vi "ReadWord.vi"(7 "Adresse":T1, 8 "error in (no error)":errorcluster, 9 "Parameter [0 ... 65535]":u16, 10 "Befehl [0 ... 65535]":u16, 11 "VISA resource name":refnum<visa-resource-name>) -> (0 "error out":errorcluster, 1 "Read Buffer":string, 2 "Regler Rückgabewert [0 ... 65535]":u16, 3 "VISA resource name out":refnum<visa-resource-name>)   [LabVIEW 2023, in "TCxxxx.lvlib"]
doc: "This VI reads a WORD value from the TCxxxx device.\n\n\nInput:\n\n- Adresse [ENUM]: this is the adress at which the function performs the read\n- Befehl [UINT16]: this is the command to the device.\n- Parameter [UINT16]: this is the parameter to read from the device (unused, always set to 0)\n\n\nOutput:\n\n- Regler Rückgabewert [UINT16]: this is the returned value of the device\n\n\n\nLast Revision: 1.0\nDate: 19.12.2016\n\nTameq Schweiz GmbH\nPeter Wilhelm\nDorfstrasse 59\nCH-5306 Tegerfelden"
uses:
  TCxxxx.lvlib
  Controls/Adresse.ctl
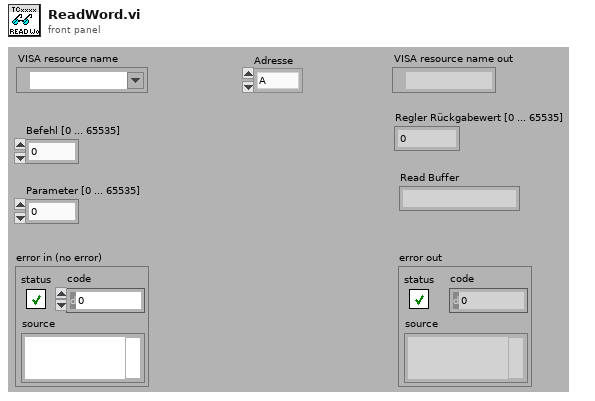
[diagram p1: front panel]
types:
  T1 = typedef "Adresse.ctl" = enum16{"A", "B", "C", "D", "E", "F", "G", "H", "I", "J", "K", "L", "M", "N", "O", "P", "Q", "R", "S", "T", "U", "V", "W", "X", "Y", "Z"}
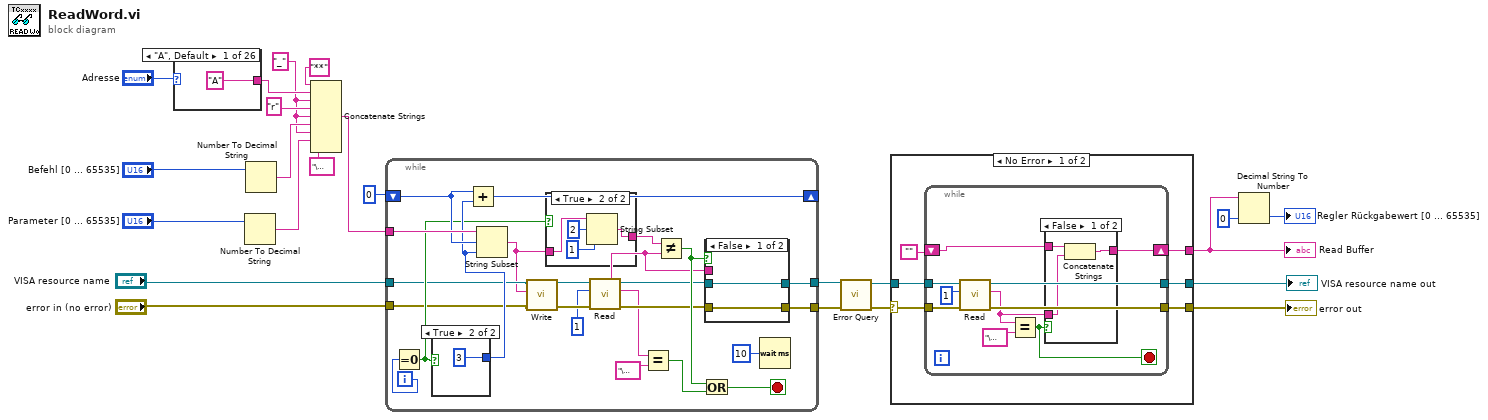
[diagram p0: block diagram]
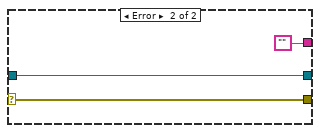
[diagram p3: hidden frame]
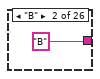
[diagram p4: hidden frame]
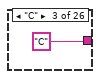
[diagram p5: hidden frame]
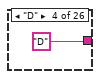
[diagram p6: hidden frame]
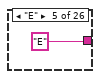
[diagram p7: hidden frame]
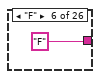
[diagram p8: hidden frame]
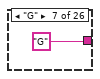
[diagram p9: hidden frame]
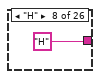
[diagram p10: hidden frame]
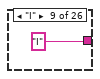
[diagram p11: hidden frame]
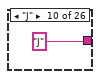
[diagram p12: hidden frame]
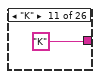
[diagram p13: hidden frame]
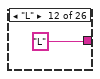
[diagram p14: hidden frame]
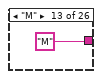
[diagram p15: hidden frame]
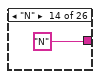
[diagram p16: hidden frame]
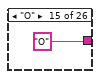
[diagram p17: hidden frame]
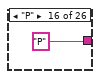
[diagram p18: hidden frame]
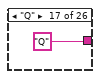
[diagram p19: hidden frame]
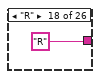
[diagram p20: hidden frame]
diagram:
  w15 = "_"
  n1 = case shown="\"A\", Default" "Adresse" {
    tunnel: ["A" "B" "C" "D" "E" "F" "G" "H" "I" "J" "K" "L" "M" "N" "O" "P" "Q" "R" "S" "T" "U" "V" "W" "X" "Y" "Z"] -> w22
    frame "A", Default {
    }
    frame "B" {
    }
    frame "C" {
    }
    frame "D" {
    }
    frame "E" {
    }
    frame "F" {
    }
    frame "G" {
    }
    frame "H" {
    }
    frame "I" {
    }
    frame "J" {
    }
    frame "K" {
    }
    frame "L" {
    }
    frame "M" {
    }
    frame "N" {
    }
    frame "O" {
    }
    frame "P" {
    }
    frame "Q" {
    }
    frame "R" {
    }
    frame "S" {
    }
    frame "T" {
    }
    frame "U" {
    }
    frame "V" {
    }
    frame "W" {
    }
    frame "X" {
    }
    frame "Y" {
    }
    frame "Z" {
    }
  }
  n2 = Number To Decimal String(number="Parameter [0 ... 65535]") -> (decimal integer string=w20:string)  [unwired: 1 in]
  n3 = Number To Decimal String(number="Befehl [0 ... 65535]") -> (decimal integer string=w21:string)  [unwired: 1 in]
  n4 = Concatenate Strings("**", w22, w15, "r", w15, w21, w15, w20, "\u0015") -> (w19:string)
  n5 = while {
    tunnel: [w61] -> w13
    tunnel: [w60] -> w14
    tunnel: "error in (no error)" -> [w57]
    tunnel: "VISA resource name" -> [w59]
    shift-right: [w67] -> _
    shift-left: 0 -> [w69]
    tunnel: w19 -> [w72]
    i -> [w70]
    stop <- w65 stop-if-true
    n6 = Equal To 0?(x=w70) -> (x = 0?=w64:bool)
    n7 = case shown="True" w64 {
      tunnel: [1 3] -> w68
      frame False {
      }
      frame True {
      }
    }
    n8 = Add(x=w69, y=w68) -> (x+y=w67:i32)
    n9 = String Subset(string=w72, offset (0)=w69, length (rest)=w68) -> (substring=w58:string)
    n10 = call "Write.vi"("error in (no error)"=w57, "Write Buffer"=w58, "VISA resource name"=w59) -> ("error out"=w55:errorcluster, "VISA resource name out"=w54:refnum<visa-resource-name>)  [unwired: 6 in, 1 out]
    n11 = case shown="True" w64 {
      tunnel: w58 -> [w80 w84]
      tunnel: [w80 w82] -> w63
      frame False {
      }
      frame True {
        n12 = String Subset(string=w84, offset (0)=2, length (rest)=1 ("length (rest)")) -> (substring=w82:string)
      }
    }
    n13 = call "Read.vi"("error in (no error)"=w55, "Byte Count"=1, "VISA resource name"=w54) -> ("error out"=w51:errorcluster, "Read Buffer"=w50:string, "VISA resource name out"=w52:refnum<visa-resource-name>)  [unwired: 5 in, 1 out]
    n14 = Equal?(x=w50, y="\u0015") -> (x = y?=w66:bool)
    n15 = Not Equal?(x=w63, y=w50) -> (x != y?=w62:bool)
    n16 = Or(x=w62, y=w66) -> (x .or. y?=w65:bool)
    n17 = case shown="False" w62 {
      tunnel: w51 -> [w74 w77]
      tunnel: [w74 w75] -> w61
      tunnel: w50 -> [_ w79]
      tunnel: w52 -> [w73 w78]
      tunnel: [w73 w76] -> w60
      frame False {
      }
      frame True {
        n18 = call "GetStatus.vi"("error in"=w77, "Status"=w79, "VISA resource name"=w78) -> ("error out"=w75:errorcluster, "VISA resource name out"=w76:refnum<visa-resource-name>)  [unwired: 7 in]
      }
    }
    n19 = Wait (ms)(milliseconds to wait=u32 10) -> ()  [unwired: 1 out]
  }
  n20 = call "Error Query.vi"("error in (no error)"=w13, "VISA resource name"=w14) -> ("error out"=w7:errorcluster, "VISA resource name out"=w6:refnum<visa-resource-name>)  [unwired: 8 in]
  n21 = case shown="No Error" w7 {
    selector: w7 -> [w91 w108]
    tunnel: w6 -> [w92 w107]
    tunnel: [w89 ""] -> w3
    tunnel: [w88 w108] -> w5
    tunnel: [w87 w107] -> w4
    frame No Error {
      n22 = while {
        tunnel: w92 -> [w100]
        tunnel: w91 -> [w99]
        shift-right: [w93] -> w89
        shift-left: "" -> [w94]
        tunnel: [w98] -> w87
        tunnel: [w97] -> w88
        stop <- w95 stop-if-true
        n23 = call "Read.vi"("error in (no error)"=w99, "Byte Count"=1, "VISA resource name"=w100) -> ("error out"=w97:errorcluster, "Read Buffer"=w96:string, "VISA resource name out"=w98:refnum<visa-resource-name>)  [unwired: 5 in, 1 out]
        n24 = Equal?(x=w96, y="\u0015") -> (x = y?=w95:bool)
        n25 = case shown="False" w95 {
          tunnel: w96 -> [w103 _]
          tunnel: w94 -> [w105 w106]
          tunnel: [w104 w106] -> w93
          frame False {
            n26 = Concatenate Strings(w105, w103) -> (w104:string)
          }
          frame True {
          }
        }
      }
    }
    frame Error {
    }
  }
  "error out" <- w5
  "VISA resource name out" <- w4
  "Read Buffer" <- w3
  n27 = Decimal String To Number(string=w3, default (0L)=u16 0 ("default (0 I32)")) -> (number=→"Regler Rückgabewert [0 ... 65535]":u16)  [unwired: 1 in, 1 out]
